vi "Servo.vi"() -> ()   [LabVIEW 2020]
doc: "This example shows how to set and read the angle of a servo.\n\nThis example expects a USB cable connected from your development PC to the Type B USB Jack (next to the power input) on the roboRIO.\n\nThis example requires the Driver Station to be running with Teleoperated Enabled."
uses:
  <vilib>/Rock Robotics/SystemInterfaces/DIO/FPGA_DIOPWMChannel.ctl
  <vilib>/Rock Robotics/SystemInterfaces/DIO/FPGA_DIOChannel.ctl
  T-Shirt Robot LV 2020/roboRIO Code/Systems/Feeder/Feeder_ACT.lvlib
panel:
  out "BAck":bool
  out "Meter":dbl(knob) scale=0.0..100.0 scale format="%.2g"
  out "error out":errorcluster
  in  "PWM Channel":T1
  in  "% of full stroke":dbl(slide) step=0.1 scale=0.0..100.0 scale format="%.2g"
  in  "stop":bool
  # "Set this input before running."
  # "PWM cable"
  # "This shows wiring for a HiTEC servo.  The black wire connects to ground (-). The red wire connects to power (V). The white or yellow wire connects to signal (S)."
  # "This example requires the Driver Station to be running with Teleoperated Enabled."
  # "The HS-785HB sail winch servo with it's large drum wheel has 3 1/2 revolutions of travel for hauling in even the largest of sails. \nWith its dual ball bearing supported output shaft the HS-785HB will provide years of reliable service."
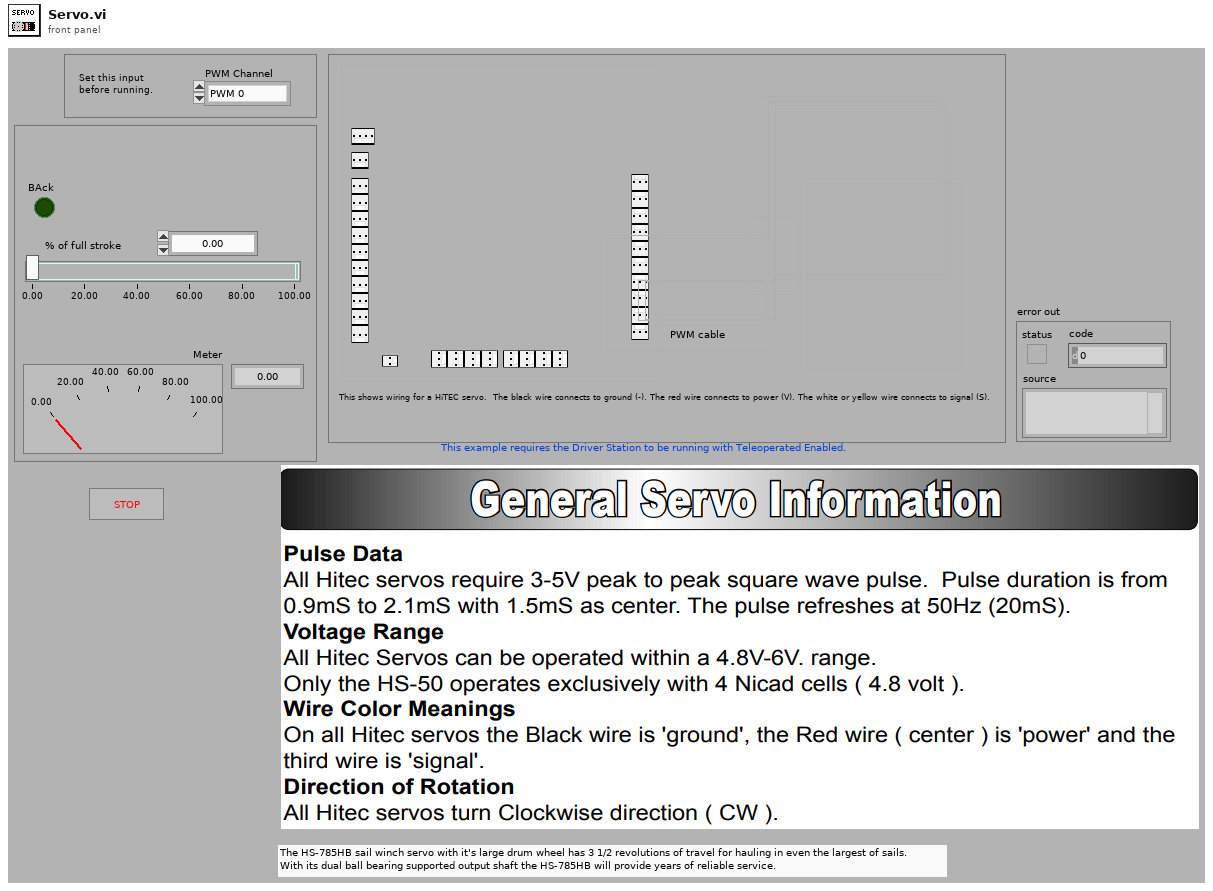
[diagram p1: front panel]
types:
  T1 = typedef "FPGA_DIOPWMChannel.ctl" = enum8{"PWM 0", "PWM 1", "PWM 2", "PWM 3", "PWM 4", "PWM 5", "PWM 6", "PWM 7", "PWM 8", "PWM 9", "PWM MXP 0", "PWM MXP 1", "PWM MXP 2", "PWM MXP 3", "PWM MXP 4", "PWM MXP 5", "PWM MXP 6", "PWM MXP 7", "PWM MXP 8", "PWM MXP 9", "Invalid"}
  T2 = typedef "FPGA_DIOChannel.ctl" = enum8{"DIO 0", "DIO 1", "DIO 2", "DIO 3", "DIO 4", "DIO 5", "DIO 6", "DIO 7", "DIO 8", "DIO 9", "DIO MXP 0", "DIO MXP 1", "DIO MXP 2", "DIO MXP 3", "DIO MXP 4", "DIO MXP 5", "DIO MXP 6", "DIO MXP 7", "DIO MXP 8", "DIO MXP 9", "DIO MXP 10", "DIO MXP 11", "DIO MXP 12", "DIO MXP 13", "DIO MXP 14", "DIO MXP 15", "SPI Port CS1", "SPI Port CS2", "SPI Port CS3", "SPI Port MISO", "SPI Port MOSI", "Invalid"}
  T3 = typedef "WPI_DigitalInputDevRef.ctl" = cluster{"DevStatus":errorcluster, "DIO Channel":T2}
  T4 = typedef "WPI_ServoDeviceRef.ctl" = cluster{"DeviceStatus":errorcluster, "PWM Channel":T1, "DeadBand":T5}
  T5 = typedef "WPI_PWMDeadband.ctl" = cluster{"Name":string, "maxPositivePwm":i32, "minPositivePwm":i32, "centerPwm":i32, "maxNegativePwm":i32, "minNegativePwm":i32, "angularRange":u16}
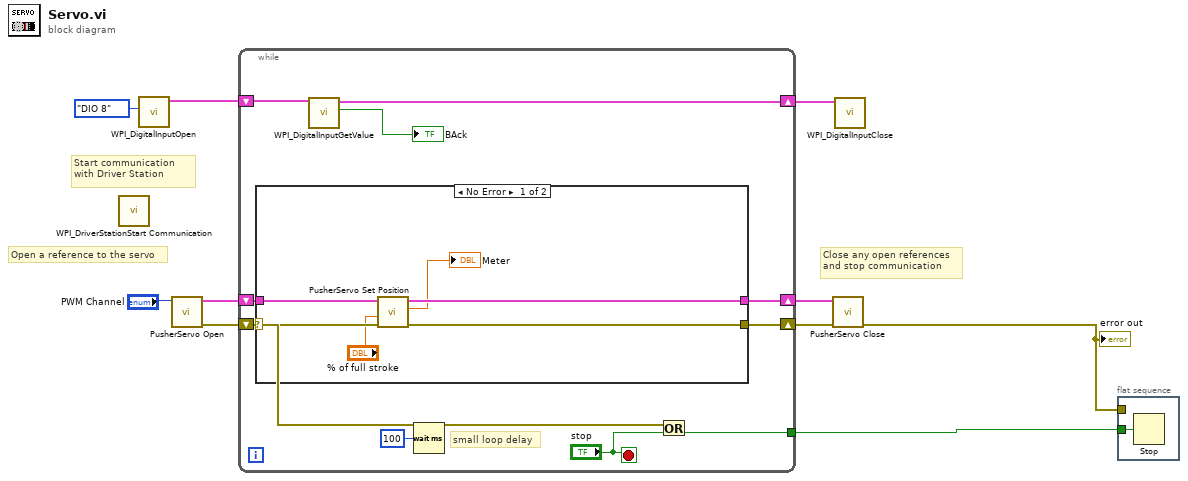
[diagram p0: block diagram]
diagram:
  # "Close any open references\nand stop communication"
  # "Start communication with Driver Station"
  # "Open a reference to the servo"
  n1 = call <vilib>:"WPI_DriverStationStart Communication.vi"() -> ()  [unwired: 3 in, 9 out]
  n2 = call <vilib>:"WPI_DigitalInputOpen.vi"("DIO Channel"=FPGA_DIOChannel."DIO 8") -> ("DigitalInputDevRef"=w3:T3)  [unwired: 9 in, 1 out]
  n3 = call "PusherServo Open.vi"("PWM Channel"="PWM Channel") -> ("Error Out"=w7:errorcluster, "ServoDeviceRef Out"=w8:T4)  [unwired: 9 in]
  n4 = while {
    tunnel: [w15] -> w10
    shift-right: [w16] -> w6
    shift-left: w7 -> [w14]
    shift-right: [w19] -> w9
    shift-left: w8 -> [w20]
    shift-right: [w12] -> w2
    shift-left: w3 -> [w13]
    stop <- "stop" stop-if-true
    # "small loop delay"
    n5 = case shown="No Error" w14 {
      selector: w14 -> [w26 w27]
      tunnel: w20 -> [w24 w28]
      tunnel: [w23 w28] -> w19
      tunnel: [w25 w27] -> w16
      frame No Error {
        n6 = call "PusherServo Set Position.vi"("Error"=w26, "Stroke (0-100)"="% of full stroke", "ServoDeviceRef"=w24) -> ("Error Out"=w25:errorcluster, "Stroke Set"=→"Meter":dbl, "ServoDeviceRef Out"=w23:T4)  [unwired: 6 in]
      }
      frame Error {
      }
    }
    n7 = call <vilib>:"WPI_DigitalInputGetValue.vi"("DigitalInputDevRef"=w13) -> ("Value"=→"BAck":bool, "DigitalInputDevRef"=w12:T3)  [unwired: 8 in, 1 out]
    n8 = Wait (ms)(milliseconds to wait=u32 100) -> ()  [unwired: 1 out]
    n9 = Or(x=w14, y="stop") -> (x .or. y?=w15:bool)
  }
  n10 = call "PusherServo Close.vi"("error in (no error)"=w6, "ServoDeviceRef Out"=w9) -> ("error out"=w5:errorcluster)  [unwired: 9 in]
  "error out" <- w5
  n11 = call <vilib>:"WPI_DigitalInputClose.vi"("DigitalInputDevRef"=w2) -> ()  [unwired: 10 in, 1 out]
  n12 = flat-sequence {
    tunnel: w10 -> [w29]
    tunnel: w5 -> [_]
    frame #0 {
      n13 = Stop(stop? (T)=w29) -> ()
    }
  }
